vi "Stop.vi"(8 "error in (no error)":errorcluster, 10 "Message in":refnum<class "StopMessage.lvclass">, 11 "BMC in":refnum<class "BMC.lvclass">) -> (0 "error out":errorcluster, 3 "BMC out":refnum<class "BMC.lvclass">)   [LabVIEW 2012, in "BMC.lvclass"]
doc: "This member function is called when the statemachine in the run.vi receives an 'stop' command. It relays the message to all observers of the component.\n\nOverride this member function in your derived class if you need additional stop functionality (but don't forget to call the parent method)."
uses:
  BMC.lvclass
  Murmex/LabVIEW/Murmex/Murmex/Murmex.lvclass
  Murmex/LabVIEW/Murmex/StopMessage/StopMessage.lvclass
panel:
  # "This method is called when the STOP\ntrigger is sent. \n\nOverride this method when your component needs to\nrespond to this trigger. \n\nCall parent for proper implementation"
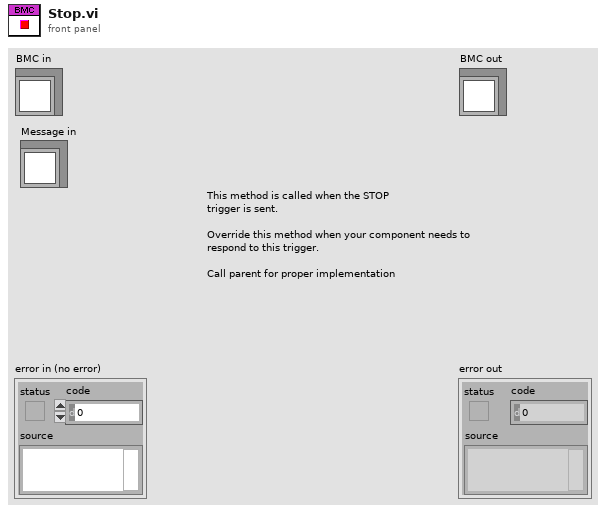
[diagram p1: front panel]
types:
  T1 = typedef "BMC.lvclass/CIUsbKub.IHostDrv.ctl" = refnum<k7>
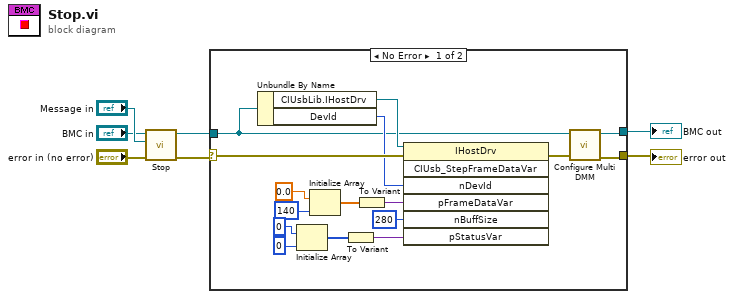
[diagram p0: block diagram]
diagram:
  n1 = call-parent "Stop.vi"("error in (no error)"="error in (no error)", "Message in"="Message in", "Murmex in"="BMC in") -> ("error out"=w4:errorcluster, "Murmex out"=w1:refnum<class "BMC.lvclass">)  [unwired: 7 in]
  n2 = case shown="No Error" w4 {
    selector: w4 -> [w14 w25]
    tunnel: [w9 w25] -> w3
    tunnel: [w8 w24] -> w2
    tunnel: w1 -> [w10 w24]
    frame No Error {
      n3 = Unbundle By Name(w10) -> ("CIUsbLib.IHostDrv"=w13:T1, "DevId"=w12:i32)
      n4 = Initialize Array(0 ("element"), 0 ("dimension size")) -> (w16:i32[])
      n5 = Initialize Array(0.0 ("element"), 140 ("dimension size")) -> (w20:dbl[])
      n6 = To Variant(anything=w16) -> (Variant=w15:variant)
      n7 = To Variant(anything=w20) -> (Variant=w22:variant)
      n8 = invoke class="IHostDrv" method="CIUsb_StepFrameDataVar"(reference=w13, error in=w14, "nDevId"=w12, "pFrameDataVar"=w22, "nBuffSize"=280, "pStatusVar"=w15) -> (error out=w11:errorcluster)  [unwired: 1 in, 6 out]
      n9 = call-dynamic "Configure Multi DMM.vi"("error in (no error)"=w11, "BMC in"=w10) -> ("error out"=w9:errorcluster, "BMC out"=w8:refnum<class "BMC.lvclass">)  [unwired: 8 in]
    }
    frame Error {
    }
  }
  "error out" <- w3
  "BMC out" <- w2
